vi "ExtendedRegisterRead.vi"(6 "Compare Bits In":T1[](array[typedef]) {"Expected Value(s)" format="%.0x"}, 7 "Extended Read/Write":T2 {"Data" format="%.0x"; "Register" format="%.0x"; "Slave Address" max=15 format="%.0x"}, 8 "error in (no error)":errorcluster, 9 "Number of Samples In":i32, 10 "Data Array":u8[][](array[numeric]), 11 "RFFE_Data In":T3 {"Toggle (high to low)" items=["0", "1", "Z", "L", "H", "X", "T", "V"]; "X Array" items=["0", "1", "Z", "L", "H", "X", "T", "V"]; "Z Array" items=["0", "1", "Z", "L", "H", "X", "T", "V"]; "L Array" items=["0", "1", "Z", "L", "H", "X", "T", "V"]; "H Array" items=["0", "1", "Z", "L", "H", "X", "T", "V"]; "One Array" items=["0", "1", "Z", "L", "H", "X", "T", "V"]; "Zero Array" items=["0", "1", "Z", "L", "H", "X", "T", "V"]}) -> (0 "error out":errorcluster, 1 "Number of Samples Out out":i32, 2 "Data Array Out":u8[][](array[numeric]), 3 "RFFE_Data Out":T3 {"Toggle (high to low)" items=["0", "1", "Z", "L", "H", "X", "T", "V"]; "X Array" items=["0", "1", "Z", "L", "H", "X", "T", "V"]; "Z Array" items=["0", "1", "Z", "L", "H", "X", "T", "V"]; "L Array" items=["0", "1", "Z", "L", "H", "X", "T", "V"]; "H Array" items=["0", "1", "Z", "L", "H", "X", "T", "V"]; "One Array" items=["0", "1", "Z", "L", "H", "X", "T", "V"]; "Zero Array" items=["0", "1", "Z", "L", "H", "X", "T", "V"]}, 4 "Compare Bits Out":T1[](array[typedef]) {"Expected Value(s)" format="%.0x"})   [LabVIEW 2013]
doc: "Builds MIPI RFFE Extended Register Read with the specified data."
uses:
  Ctrls/RFFE_Data.ctl
  Ctrls/ClockDataChannels.ctl
  Ctrls/ExtendedRegReadWrite.ctl
  Ctrls/ReadInfo.ctl
  Ctrls/Commands.ctl
  Ctrls/Read_Write_Data.ctl
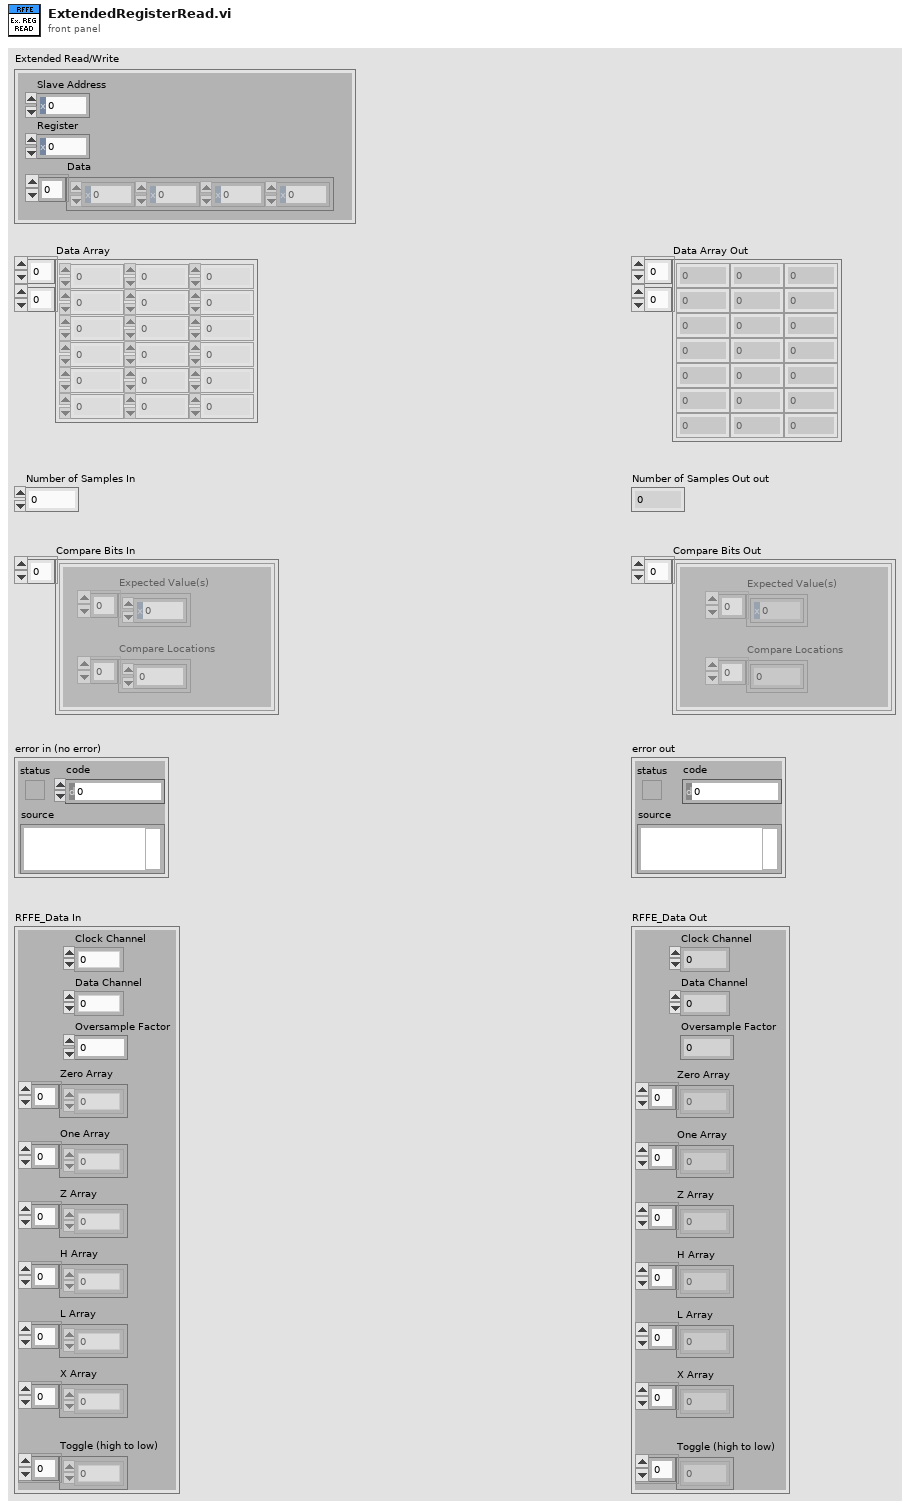
[diagram p1: front panel]
types:
  T1 = typedef "ReadInfo.ctl" = cluster{"Expected Value(s)":u8[], "Compare Locations":u32[]}
  T2 = typedef "ExtendedRegReadWrite.ctl" = cluster{"Slave Address":u8, "Register":u8, "Data":u8[]}
  T3 = typedef "RFFE_Data.ctl" = cluster{"Clock Channel":T4, "Data Channel":T4, "Oversample Factor":u8, "Zero Array":u8[], "One Array":u8[], "Z Array ":u8[], "H Array":u8[], "L Array":u8[], "X Array":u8[], "Toggle (high to low)":u8[]}
  T4 = typedef "ClockDataChannels.ctl" = enum16{"0", "1"}
  T5 = typedef "Read_Write_Data.ctl" = cluster{"Data":u8, "Read/Write":enum16{"Read", "Write"}}
  T6 = typedef "Commands.ctl" = cluster{"Command":enum16{"Extended Register Write", "Extended Register Read", "Extended Register Write Long", "Extended Register Read Long", "Register Write", "Register Read", "Register 0 Write"}, "Data/Address/ByteCount":u8}
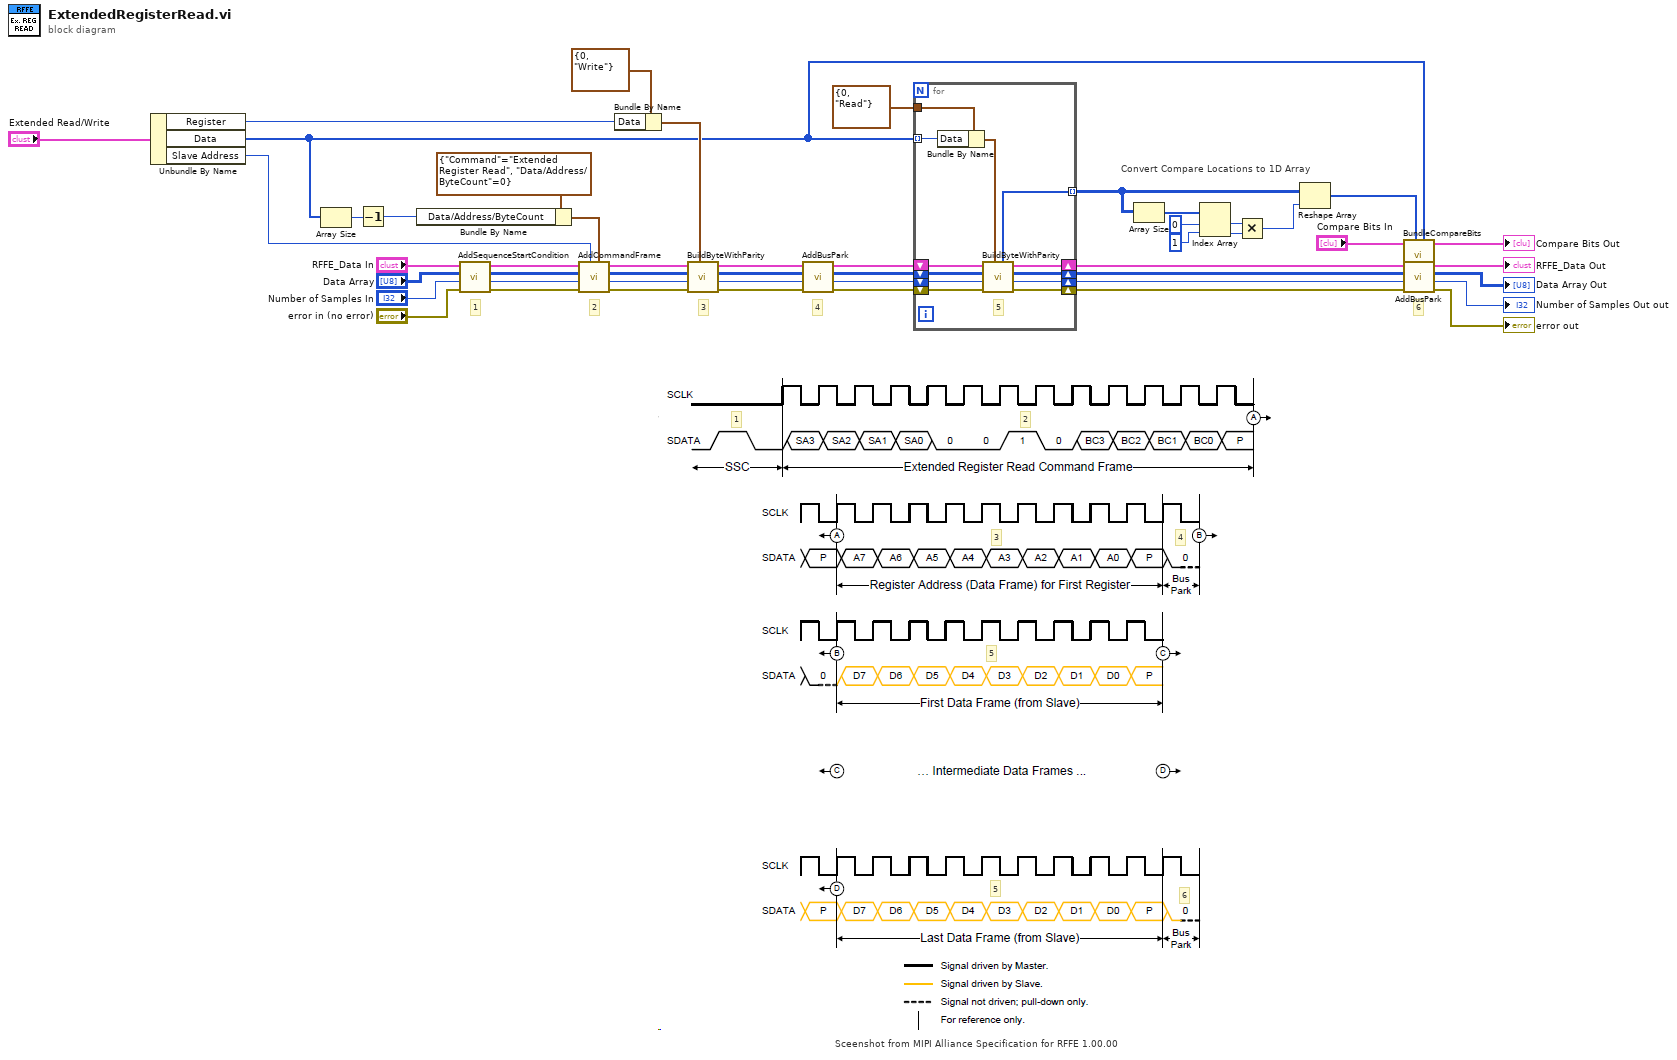
[diagram p0: block diagram]
diagram:
  # "5"
  # "Sceenshot from MIPI Alliance Specification for RFFE 1.00.00"
  # "Convert Compare Locations to 1D Array"
  # "6"
  # "5"
  # "4"
  # "3"
  # "2"
  # "1"
  # "6"
  # "4"
  # "3"
  # "2"
  # "1"
  n1 = Unbundle By Name("Extended Read/Write") -> ("Register"=w14:u8, "Data"=w13:u8[], "Slave Address"=w18:u8)
  n2 = Array Size(array=w13) -> (size(s)=w31:i32)
  n3 = Decrement(x=w31) -> (x-1=w28:i32)
  n4 = Bundle By Name(cluster=T6 {"Command"=enum."Extended Register Read", "Data/Address/ByteCount"=0} ("Command"), "Data/Address/ByteCount"=w28) -> (w19:T6)
  n5 = call "AddSequenceStartCondition.vi"("error in (no error)"="error in (no error)", "Number of Samples In"="Number of Samples In", "Data Array In"="Data Array", "RFFE_Data In"="RFFE_Data In") -> ("error out"=w41:errorcluster, "Number of Samples Out"=w47:i32, "Data Array Out"=w42:u8[][], "RFFE_Data Out"=w43:T3)  [unwired: 4 in]
  n6 = call "AddCommandFrame.vi"("Command"=w19, "Slave Address"=w18, "error in (no error)"=w41, "Number of Samples In"=w47, "Data Array In"=w42, "RFFE_Data"=w43) -> ("error out"=w44:errorcluster, "Number of Samples Out"=w20:i32, "Data Array Out"=w21:u8[][], "Configuratation Out"=w45:T3)  [unwired: 2 in]
  n7 = Bundle By Name(cluster=T5 {"Data"=0, "Read/Write"=enum."Write"} ("Read/Write Data"), "Data"=w14) -> (w29:T5)
  n8 = call "BuildByteWithParity.vi"("Read/Write Data"=w29, "error in"=w44, "Number of Samples In"=w20, "Data Array In"=w21, "RFFE_Data In"=w45) -> ("error out"=w24:errorcluster, "Number of Samples Out"=w22:i32, "Data Array Out"=w23:u8[][], "RFFE_Data Out"=w25:T3)  [unwired: 2 in, 1 out]
  n9 = call "AddBusPark.vi"("error in (no error)"=w24, "Number of Samples In"=w22, "Data Array In"=w23, "RFFE_Data In"=w25) -> ("error out"=w26:errorcluster, "Number of Samples Out"=w15:i32, "Data Array Out"=w16:u8[][], "RFFE_Data Out"=w17:T3)  [unwired: 4 in]
  n10 = for {
    shift-right: [w60] -> w34
    shift-left: w26 -> [w61]
    shift-right: [w57] -> w32
    shift-left: w15 -> [w59]
    shift-right: [w56] -> w33
    shift-left: w16 -> [w58]
    shift-right: [w55] -> w4
    shift-left: w17 -> [w54]
    tunnel: w13 -> [w53] mode=indexing
    tunnel: T5 {"Data"=0, "Read/Write"=enum."Read"} ("Read/Write Data") -> [w51]
    tunnel: [w50] -> w7 mode=indexing
    # "5"
    n11 = Bundle By Name(cluster=w51, "Data"=w53) -> (w52:T5)
    n12 = call "BuildByteWithParity.vi"("Read/Write Data"=w52, "error in"=w61, "Number of Samples In"=w59, "Data Array In"=w58, "RFFE_Data In"=w54) -> ("error out"=w60:errorcluster, "Number of Samples Out"=w57:i32, "Data Array Out"=w56:u8[][], "RFFE_Data Out"=w55:T3, "Compare Locations"=w50:u32[])  [unwired: 2 in]
  }
  n13 = Array Size(array=w7) -> (size(s)=w8:i32[])
  n14 = Index Array(array=w8, index #1=0 ("index"), index #2=1 ("index")) -> (element #1=w9:i32, element #2=w5:i32)
  n15 = Multiply(x=w9, y=w5) -> (x*y=w10:i32)
  n16 = Reshape Array(w7, w10) -> (w6:u32[])
  n17 = call "BundleCompareBits.vi"("Expected Value(s)"=w13, "Compare Locations"=w6, "Compare Bits In"="Compare Bits In") -> ("Compare Bits Out"=→"Compare Bits Out":T1[])  [unwired: 8 in]
  n18 = call "AddBusPark.vi"("error in (no error)"=w34, "Number of Samples In"=w32, "Data Array In"=w33, "RFFE_Data In"=w4) -> ("error out"=→"error out":errorcluster, "Number of Samples Out"=→"Number of Samples Out out":i32, "Data Array Out"=→"Data Array Out":u8[][], "RFFE_Data Out"=→"RFFE_Data Out":T3)  [unwired: 4 in]
